vi "Processing.IsRunning.vi"(8 "error in (no error)":errorcluster) -> (0 "error out":errorcluster, 2 "running?":bool)   [LabVIEW 2019, in "Tools.lvlib"]
uses:
  Tools.lvlib
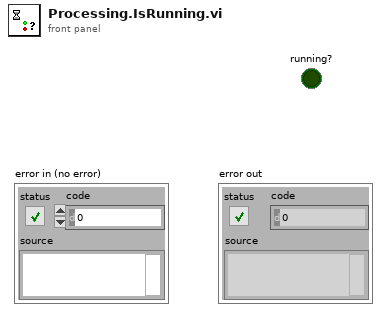
[diagram p1: front panel]
types:
  T1 = enum32{"Bad", "Idle", "Run top level", "Running"}
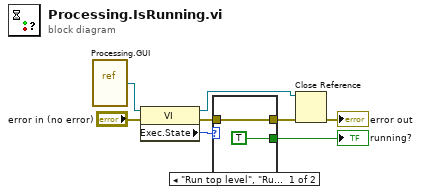
[diagram p0: block diagram]
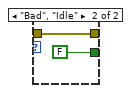
[diagram p2: hidden frame]
diagram:
  n1 = vi-ref "Processing.GUI.vi"() -> (w7:refnum<vi>)
  n2 = property class="VI"(reference=w7, error in="error in (no error)") -> (reference out=w6:refnum<vi>, error out=w2:errorcluster, "Exec.State"=w4:T1)
  n3 = case shown="\"Run top level\", \"Running\"" w4 {
    tunnel: [TRUE FALSE] -> w3
    tunnel: w2 -> [w9 w11]
    tunnel: [w9 w11] -> w1
    frame "Run top level", "Running" {
    }
    frame "Bad", "Idle" {
    }
  }
  "running?" <- w3
  n4 = Close Reference(reference=w6, error in (no error)=w1) -> (error out=→"error out":errorcluster)
